vi "Jacobian Stiffness Column 2 Record.vi"(9 "Step":string, 10 "Jacobian Stiffness Column":T1, 11 "Time Stamp":timestamp) -> (2 "Record":string)   [LabVIEW 2009]
uses:
  Global Data/Jacobian Stiffness Column.ctl
  Global Data/Jacobian Stiffness Column Id.ctl
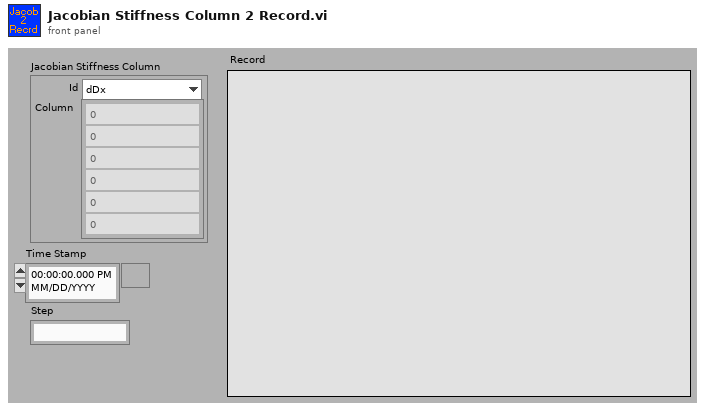
[diagram p1: front panel]
types:
  T1 = typedef "Jacobian Stiffness Column.ctl" = cluster{"Id":T2, "Column":dbl[]}
  T2 = typedef "Jacobian Stiffness Column Id.ctl" = enum16{"dDx", "dDy", "dDz", "dRx", "dRy", "dRz"}
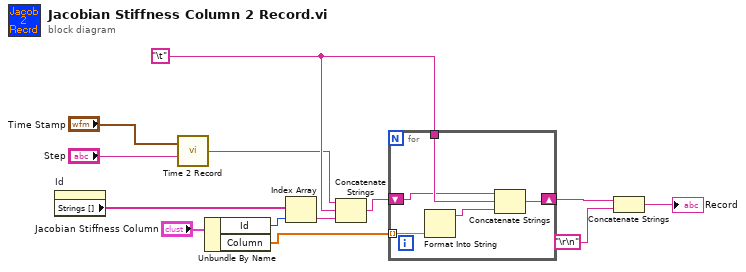
[diagram p0: block diagram]
diagram:
  w4 = "\t"
  n1 = property on="Id" class="Enum (strict)"() -> ("Strings []"=w10:string[])  [unwired: 2 in, 2 out]
  n2 = call "Time 2 Record.vi"("Step"="Step", "Time Stamp"="Time Stamp") -> ("String"=w3:string)
  n3 = Unbundle By Name("Jacobian Stiffness Column") -> ("Id"=w11:T2, "Column"=w12:dbl[])
  n4 = Index Array(array=w10, index=w11) -> (element=w9:string)
  n5 = Concatenate Strings(w3, w4, w9) -> (w5:string)
  n6 = for {
    tunnel: w12 -> [w18] mode=indexing
    tunnel: w4 -> [w16]
    shift-right: [w15] -> w8
    shift-left: w5 -> [w14]
    n7 = Format Into String(w18) -> (resulting string=w17:string)  [unwired: 3 in, 1 out]
    n8 = Concatenate Strings(w14, w16, w17) -> (w15:string)
  }
  n9 = Concatenate Strings(w8, "\r\n") -> (→"Record":string)
